vi "svfa_Spectrum Peak Search.vi"(8 "error in (no error)":errorcluster, 9 "peak search settings":T2 {"Threshold" format="%.2f"}, 10 "spectral info":T1, 11 "spectrum":cluster{"f0":dbl, "df":dbl, "spectrum":dbl[]}={"f0"=1.0, "df"=1.0, "spectrum"=[]} {"spectrum" format="%.2f"; "df" format="%.2f"; "f0" format="%.2f"}) -> (0 "error out":errorcluster, 2 "# of peaks":i32, 3 "peaks":cluster{"frequency":dbl, "Value":dbl}[](array[cluster]) {"Value" format="%.2f"; "frequency" format="%.2f"})   [LabVIEW 2017]
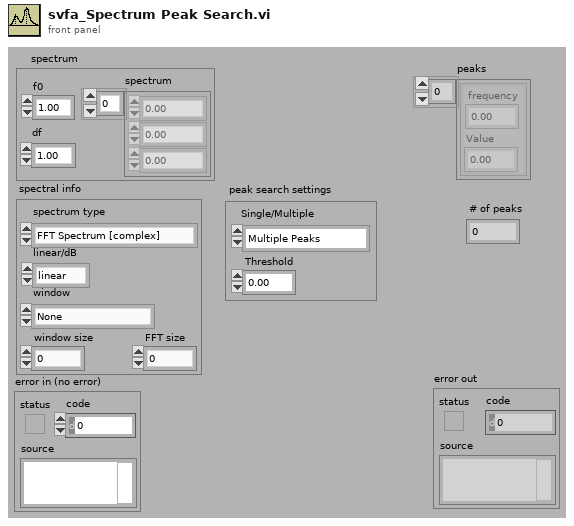
[diagram p1: front panel]
types:
  T1 = cluster{"spectrum type":enum16{"FFT Spectrum [complex]", "Amplitude [Magnitude]", "Power [Magnitude^2]", "Cross Spectrum [complex]", "Frequency Response [Complex]"}, "linear/dB":enum16{"linear", "dB"}, "window":enum16{"None ", "Hanning", "Hamming", "Blackman-Harris", "Exact Blackman", "Blackman", "Flat Top", "4 Term B-Harris ", "7 Term B-Harris", "Low Sidelobe"}, "window size":i32, "FFT size":i32}
  T2 = cluster{"Single/Multiple":enum16{"Multiple Peaks", "Single Max Peak"}, "Threshold":dbl}
  T3 = enum16{"FFT Spectrum [complex]", "Amplitude [Magnitude]", "Power [Magnitude^2]", "Cross Spectrum [complex]", "Frequency Response [Complex]"}
  T4 = enum16{"None ", "Hanning", "Hamming", "Blackman-Harris", "Exact Blackman", "Blackman", "Flat Top", "4 Term B-Harris ", "7 Term B-Harris", "Low Sidelobe"}
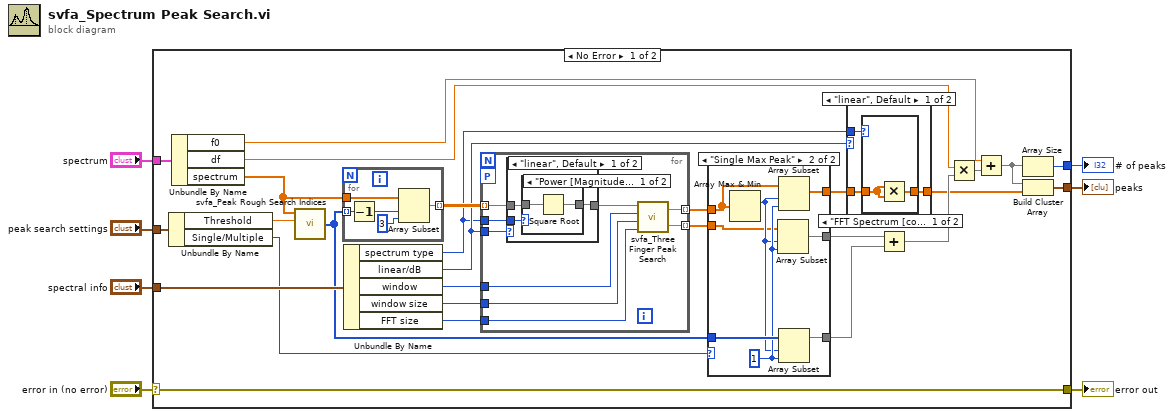
[diagram p0: block diagram]
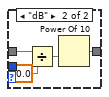
[diagram p3: hidden frame]
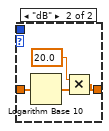
[diagram p5: hidden frame]
diagram:
  n1 = case shown="No Error" "error in (no error)" {
    selector: "error in (no error)" -> [w33 w80]
    tunnel: "spectral info" -> [w34 _]
    tunnel: [w33 w80] -> w6
    tunnel: [w32 _] -> w4
    tunnel: [w31 _] -> w3
    tunnel: "peak search settings" -> [w30 _]
    tunnel: "spectrum" -> [w21 _]
    frame No Error {
      n2 = Unbundle By Name(w30) -> ("Threshold"=w26:dbl, "Single/Multiple"=w8:enum16{"Multiple Peaks", "Single Max Peak"})
      n3 = Unbundle By Name(w21) -> ("f0"=w20:dbl, "df"=w19:dbl, "spectrum"=w11:dbl[])
      n4 = call <vilib>:"svfa_Peak Rough Search Indices.vi"("x"=w11, "threshold"=w26) -> ("peak indices"=w18:i32[])  [unwired: 3 in]
      n5 = for {
        tunnel: w18 -> [w76] mode=indexing
        tunnel: w11 -> [w79]
        tunnel: [w75] -> w12 mode=indexing
        n6 = Decrement(x=w76) -> (x-1=w77:i32)
        n7 = Array Subset(array=w79, index=w77, length=3 ("Array Length")) -> (w75:dbl[])
      }
      n8 = Unbundle By Name(w34) -> ("spectrum type"=w9:T3, "linear/dB"=w10:enum16{"linear", "dB"}, "window"=w15:T4, "window size"=w14:i32, "FFT size"=w13:i32)
      n9 = for {
        tunnel: w15 -> [w43]
        tunnel: w14 -> [w42]
        tunnel: w13 -> [w41]
        tunnel: [w40] -> w17 mode=indexing
        tunnel: [w39] -> w16 mode=indexing
        workers-P: _ -> [_]
        tunnel: w12 -> [w36] mode=indexing
        tunnel: w10 -> [w38]
        tunnel: w9 -> [w37]
        n10 = case shown="\"linear\", Default" w38 {
          tunnel: w36 -> [w46 w53]
          tunnel: [w45 w52] -> w35
          tunnel: w37 -> [w44 _]
          frame "linear", Default {
            n11 = case shown="\"Power [Magnitude^2]\", Default" w44 {
              tunnel: w46 -> [w48 w49]
              tunnel: [w47 w49] -> w45
              frame "Power [Magnitude^2]", Default {
                n12 = Square Root(x=w48) -> (sqrt(x)=w47:dbl[])
              }
              frame "Amplitude [Magnitude]" {
              }
            }
          }
          frame "dB" {
            n13 = Divide(x=w53, y=20.0 ("x")) -> (x/y=w50:dbl[])
            n14 = Power Of 10(x=w50) -> (10^x=w52:dbl[])
          }
        }
        n15 = call <vilib>:"svfa_Three Finger Peak Search.vi"("FFT Size"=w41, "window length"=w42, "window"=w43, "three fingers"=w35) -> ("freq"=w39:dbl, "amplitude"=w40:dbl)
      }
      n16 = case shown="\"Single Max Peak\"" w8 {
        tunnel: w17 -> [w66 w74]
        tunnel: [w66 w72] -> w28
        tunnel: w16 -> [w65 w67]
        tunnel: [w65 w73] -> w23
        tunnel: w18 -> [w64 w71]
        tunnel: [w64 w68] -> w22
        frame "Multiple Peaks", Default {
        }
        frame "Single Max Peak" {
          w70 = 1 ("Array Length")
          n17 = Array Max & Min(array=w74) -> (max index (indices)=w69:i32)  [unwired: 3 out]
          n18 = Array Subset(array=w67, index=w69, length=w70) -> (w73:dbl[])
          n19 = Array Subset(array=w74, index=w69, length=w70) -> (w72:dbl[])
          n20 = Array Subset(array=w71, index=w69, length=w70) -> (w68:i32[])
        }
      }
      n21 = case shown="\"linear\", Default" w10 {
        tunnel: w28 -> [w56 w63]
        tunnel: [w55 w62] -> w24
        tunnel: w9 -> [w54 _]
        frame "linear", Default {
          n22 = case shown="\"FFT Spectrum [complex]\", Default" w54 {
            tunnel: w56 -> [w57 w59]
            tunnel: [w58 w59] -> w55
            frame "FFT Spectrum [complex]", Default {
              n23 = Multiply(x=w57, y=w57) -> (x*y=w58:dbl[])
            }
            frame "Amplitude [Magnitude]" {
            }
          }
        }
        frame "dB" {
          n24 = Logarithm Base 10(1:w63) -> (0:w61:dbl[])
          n25 = Multiply(x=20.0, y=w61) -> (x*y=w62:dbl[])
        }
      }
      n26 = Add(x=w23, y=w22) -> (x+y=w27:dbl[])
      n27 = Multiply(x=w19, y=w27) -> (x*y=w29:dbl[])
      n28 = Add(x=w20, y=w29) -> (x+y=w25:dbl[])
      n29 = Array Size(array=w25) -> (size(s)=w31:i32)
      n30 = Build Cluster Array ("Index & Bundle Cluster Array")(w25, w24) -> (w32:cluster{dbl, "amplitude":dbl}[])
    }
    frame Error {
    }
  }
  "error out" <- w6
  "peaks" <- w4
  "# of peaks" <- w3
